vi "test Abort All numeric.vi"(11 "Test Case In":refnum<class "Tests Event MessengerM.lvclass">) -> (0 "error out":errorcluster, 3 "Test Case Out":refnum<class "Tests Event MessengerM.lvclass">)   [LabVIEW 2020, in "Tests Event MessengerM.lvclass"]
uses:
  Tests Event MessengerM.lvclass
  C:/Program Files/National Instruments/LabVIEW 2025/vi.lib/Astemes/LUnit/Test Case.lvclass
  <vilib>/Astemes/LUnit/Test Case.lvclass/Test Case.ctl
  <vilib>/Astemes/LUnit/Test Case.lvclass
  <extravilib>/ChannelInstances/Event MessengerM-i32.lvlib
panel:
  out "msg 2":i32
  out "msg":i32
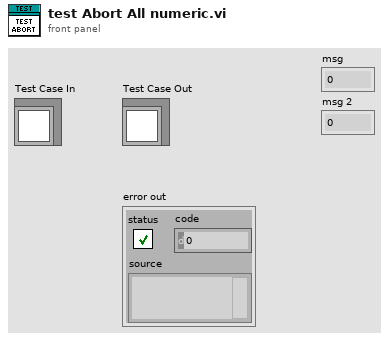
[diagram p1: front panel]
types:
  T1 = typedef "Event MessengerM-i32.lvlib/))Channel.ctl" = refnum<queue>
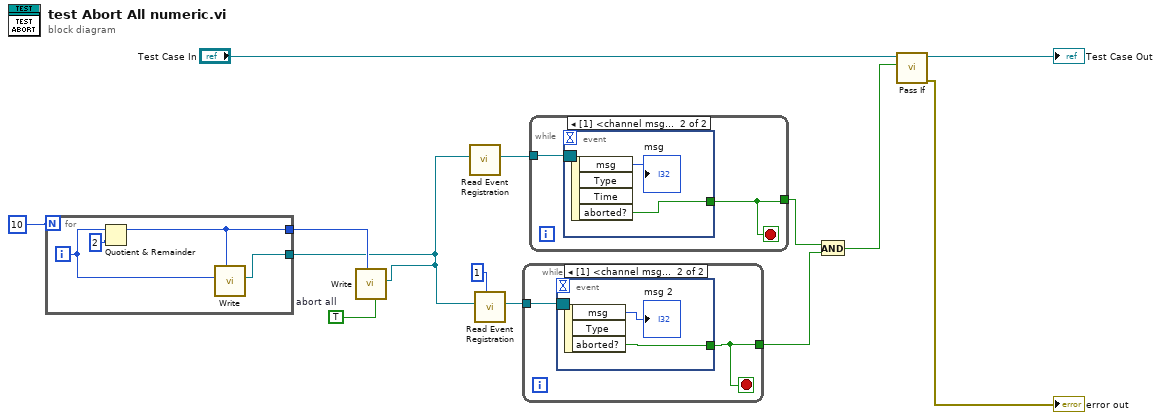
[diagram p0: block diagram]
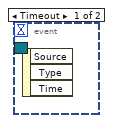
[diagram p2: hidden frame]
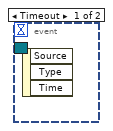
[diagram p3: hidden frame]
diagram:
  w6 = TRUE  # abort all
  n1 = for {
    N: 10 -> [_]
    tunnel: [w16] -> w4
    tunnel: [w14] -> w5
    i -> [w15]
    n2 = Quotient & Remainder(x=w15, y=2) -> (x-y*floor(x/y)=w14:i32)  [unwired: 1 out]
    n3 = call <extravilib>:"Write.vi"("subchannel (0)"=w14, "element"=w15) -> ("channel"=w16:T1)  [unwired: 8 in, 1 out]
  }
  n4 = call <extravilib>:"Write.vi"("channel"=w4, "abort all (F)"=w6, "subchannel (0)"=w5) -> ()  [unwired: 8 in, 1 out]
  n5 = call <extravilib>:"Read Event Registration.vi"("channel"=w4) -> ("event registration refnum"=w3:refnum<event-registration>)  [unwired: 10 in]
  n6 = call <extravilib>:"Read Event Registration.vi"("subchannel (0)"=1, "channel"=w4) -> ("event registration refnum"=w2:refnum<event-registration>)  [unwired: 9 in]
  n7 = while {
    tunnel: w2 -> [w19]
    tunnel: [w18] -> w8
    stop <- w18 stop-if-true
    n8 = event shown="[1] <channel msg>: User Event" {
      selector: w19 -> [_ _]
      dyn-events: _ -> [_ _]
      timeout: _ -> [_ _]
      tunnel: [_ w21] -> w18
      event Timeout {
        n9 = event-data() -> ()  [unwired: 1 in, 3 out]
      }
      event User Event {
        n10 = event-data() -> ("msg"=→"msg 2":i32, "aborted?"=w21:bool)  [unwired: 1 in, 1 out]
      }
    }
  }
  n11 = while {
    tunnel: w3 -> [w23]
    tunnel: [w22] -> w7
    stop <- w22 stop-if-true
    n12 = event shown="[1] <channel msg>: User Event" {
      selector: w23 -> [_ _]
      dyn-events: _ -> [_ _]
      timeout: _ -> [_ _]
      tunnel: [_ w25] -> w22
      event Timeout {
        n13 = event-data() -> ()  [unwired: 1 in, 3 out]
      }
      event User Event {
        n14 = event-data() -> ("msg"=→"msg":i32, "aborted?"=w25:bool)  [unwired: 1 in, 2 out]
      }
    }
  }
  n15 = And(x=w7, y=w8) -> (x .and. y?=w9:bool)
  n16 = call <vilib>:"Pass If.vi"("Pass?"=w9, "LUnit Test Case In"="Test Case In") -> ("error out"=→"error out":errorcluster, "LUnit Test Case Out"=→"Test Case Out":refnum<class "Tests Event MessengerM.lvclass">)  [unwired: 8 in]
